vi "ProtocolSetting_SubVI.vi"(11 "selected path":path) -> (2 "all rows":string[](array[string]), 3 "whole match":string)   [LabVIEW 2014]
uses:
  <vilib>/Utility/file.llb/Read From Spreadsheet File (string).vi
  <vilib>/regexp/Match Regular Expression.xnode
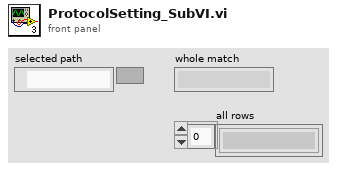
[diagram p1: front panel]
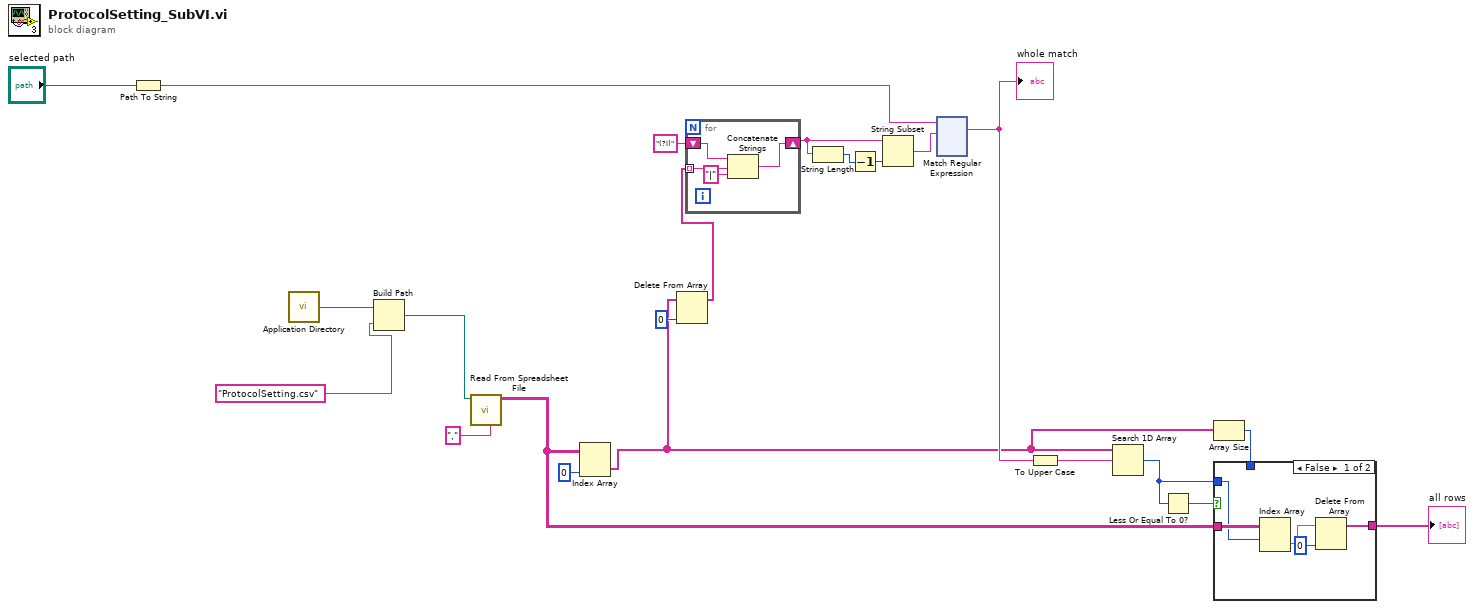
[diagram p0: block diagram]
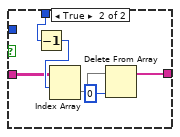
[diagram p2: hidden frame]
diagram:
  n1 = Path To String(path="selected path") -> (string=w8:string)
  n2 = call <vilib>:"Application Directory.vi"() -> ("Application Directory"=w5:path)
  n3 = Build Path(base path=w5, name or relative path="ProtocolSetting.csv" ("file path (dialog if empty)")) -> (appended path=w6:path)
  n4 = call-poly <vilib>:"Read From Spreadsheet File.vi"("delimiter (\\t)"="," ("delimiter (\\t)"), "file path (dialog if empty)"=w6) -> ("all rows"=w21:string[][])  [unwired: 5 in, 4 out]
  n5 = Index Array(array=w21, index (col)=0 ("disabled index (col)")) -> (element=w2:string[])  [unwired: 1 in]
  n6 = Delete From Array(array=w2, index=0) -> (array with subset deleted=w18:string[])  [unwired: 1 in, 1 out]
  n7 = for {
    shift-right: [w25] -> w9
    shift-left: "(?i)" -> [w26]
    tunnel: w18 -> [w24] mode=indexing
    n8 = Concatenate Strings(w26, w24, "|" ("string")) -> (w25:string)
  }
  n9 = String Length(string=w9) -> (length=w11:i32)
  n10 = Decrement(x=w11) -> (x-1=w10:i32)
  n11 = String Subset(string=w9, length (rest)=w10) -> (substring=w16:string)  [unwired: 1 in]
  n12 = xnode "Match Regular Expression"("input string"=w8, "regular expression"=w16) -> ("whole match"=w19:string)  [unwired: 4 in, 4 out]
  "whole match" <- w19
  n13 = To Upper Case(1:w19) -> (0:w20:string)
  n14 = Search 1D Array(1D array=w2, element=w20) -> (index of element=w3:i32)  [unwired: 1 in]
  n15 = Less Or Equal To 0?(x=w3) -> (x <= 0?=w4:bool)
  n16 = Array Size(array=w2) -> (size(s)=w1:i32)
  n17 = case shown="False" w4 {
    tunnel: [w31 w36] -> w22
    tunnel: w21 -> [w28 w32]
    tunnel: w3 -> [w27 _]
    tunnel: w1 -> [_ w35]
    frame False {
      n18 = Index Array(array=w28, index (row)=w27) -> (element=w29:string[])  [unwired: 1 in]
      n19 = Delete From Array(array=w29, index=0) -> (array with subset deleted=w31:string[])  [unwired: 1 in, 1 out]
    }
    frame True {
      n20 = Decrement(x=w35) -> (x-1=w34:i32)
      n21 = Index Array(array=w32, index (row)=w34) -> (element=w33:string[])  [unwired: 1 in]
      n22 = Delete From Array(array=w33, index=0) -> (array with subset deleted=w36:string[])  [unwired: 1 in, 1 out]
    }
  }
  "all rows" <- w22
